vi "P3 E1 RLJ 2015640305.vi"() -> ()   [LabVIEW 2016]
doc: "practica 3: ESTRUCTURAS DE CONTROL\nEjercicio 1 (Cajero automatico).\nNOMBRE DEL ARCHIVO: P3 E1 RLJ 2015640305.vi.\nALUMNO:Ramirez Lopez Jesus Alberto"
uses:
  State.ctl
  Data.ctl
  Control 3.ctl
panel:
  in  "IR A MENU":bool
  in  "Exit":bool
  out "Tab":T1(tab)
  in  "id":bool
  out "Boolean":bool
  out "Pict Ring":i32(ring)
  in  "ok":bool
  in  "0":bool
  in  "8":bool
  in  "9":bool
  in  "7":bool
  in  "6":bool
  in  "5":bool
  in  "4":bool
  in  "3":bool
  in  "2":bool
  in  "1":bool
  out "concatenated string 2":string
  in  "s 2":bool
  out "String 3":string
  in  "edo de cuenta":bool
  in  "deposito oc":bool
  in  "donativo":bool
  in  "pago de tiempo aire":bool
  in  "pago de tarjeta":bool
  in  "retiro":bool
  in  "SALIR":bool
  in  "ingresar":bool
  out "String":string
  in  "Numeric Control 2":dbl
  in  "abonar":bool
  in  "Numeric Control":dbl
  out "String 2":string
  out "Array 2":bool[](array[boolean])
  in  "100":bool
  in  "200":bool
  in  "300":bool
  in  "500":bool
  out "String 4":string
  in  "CDH Tepeyac":bool
  in  "CILAS":bool
  in  "ALAMPYME":bool
  in  "nicolasa":bool
  out "String 6":string
  in  "pedro":bool
  in  "juan":bool
  out "concate":string
  in  "ok 2":bool
  in  "s 3":bool
  in  "1 2":bool
  in  "2 2":bool
  in  "3 2":bool
  in  "4 2":bool
  in  "5 2":bool
  in  "6 2":bool
  in  "7 2":bool
  in  "9 2":bool
  in  "8 2":bool
  in  "0 2":bool
  out "String 7":string
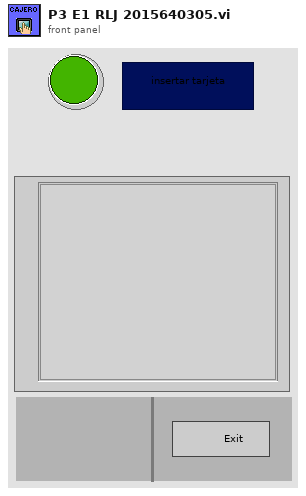
[diagram p1: front panel]
types:
  T1 = enum32{"Page 1", "Page 2", "Page 3", "Page 4", "Page 5", "Page 6", "Page 7", "Page 8", "Page 9", "Page 10"}
  T2 = typedef "Data.ctl" = cluster{"true/false":bool, "String 1":string, "saldo":dbl, "deuda":dbl, "id":bool, "pag1":bool, "seleccion":bool, "edo de cuentas":string, "cuenta error":dbl}
  T3 = typedef "State.ctl" = enum16{"Initialize", "Wait for Event", "id", "contraseña", "error", "retiro de efectivo", "pago de tarjeta", "compra de tiempo aire", "estado de cuenta", "donativo", "deposito a otra cuentas", "teclado", "menu", "Exit"}
  T4 = typedef "Control 3.ctl" = enum32{"Page 1", "Page 2", "Page 3", "Page 4", "Page 5", "Page 6", "Page 7", "Page 8", "Page 9", "Page 10"}
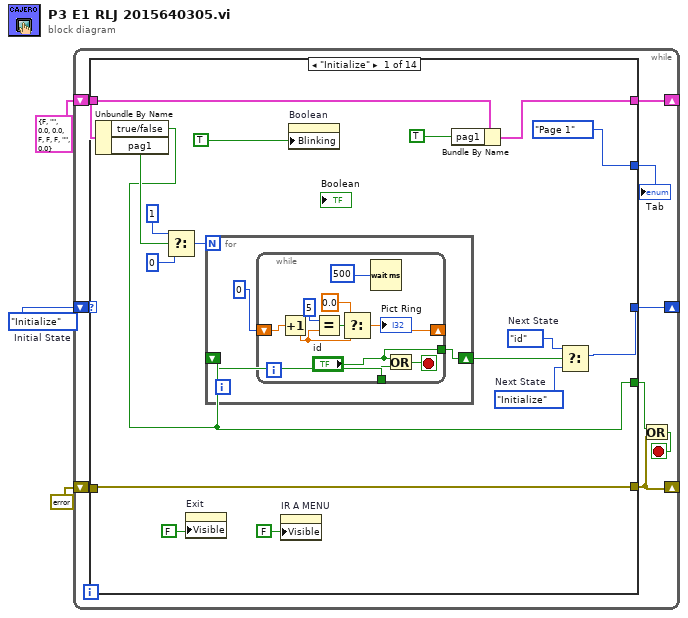
[diagram p0: block diagram]
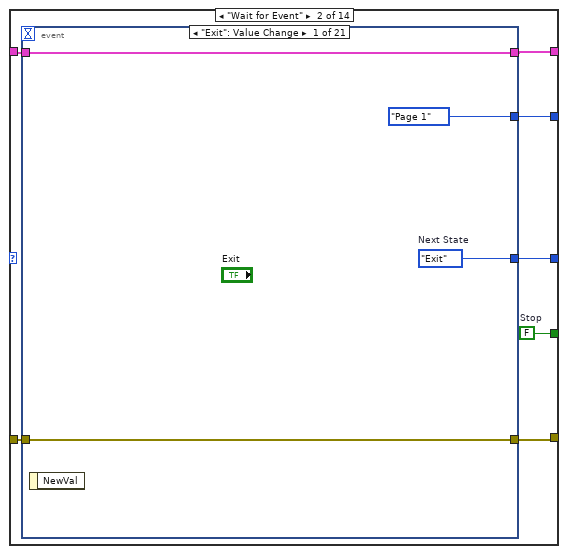
[diagram p2: hidden frame]
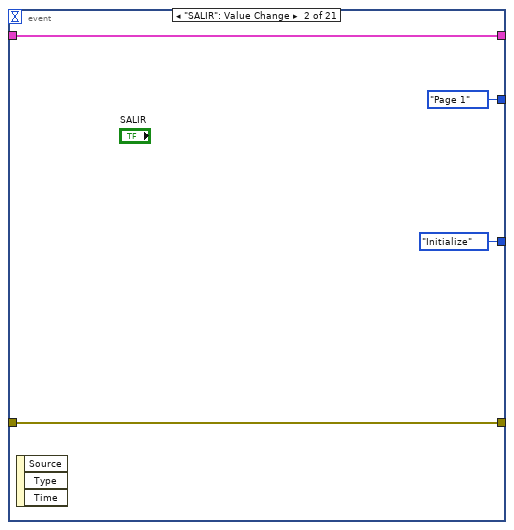
[diagram p3: hidden frame]
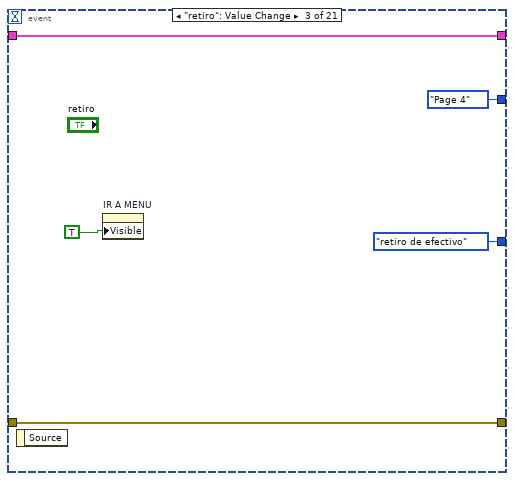
[diagram p4: hidden frame]
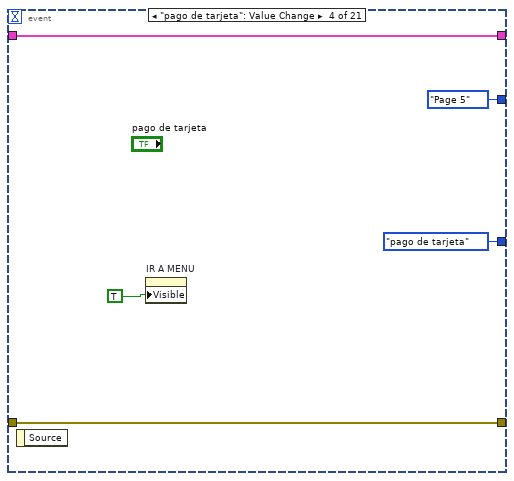
[diagram p5: hidden frame]
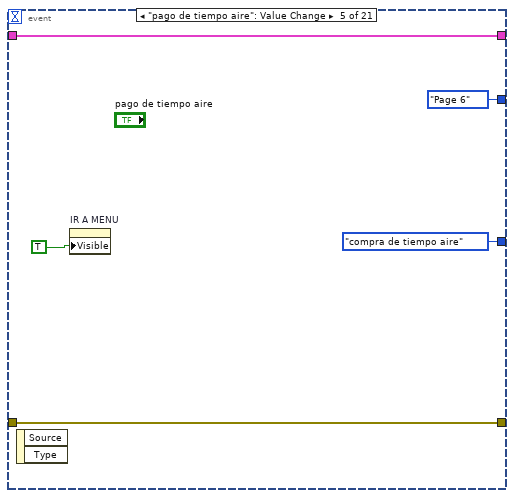
[diagram p6: hidden frame]
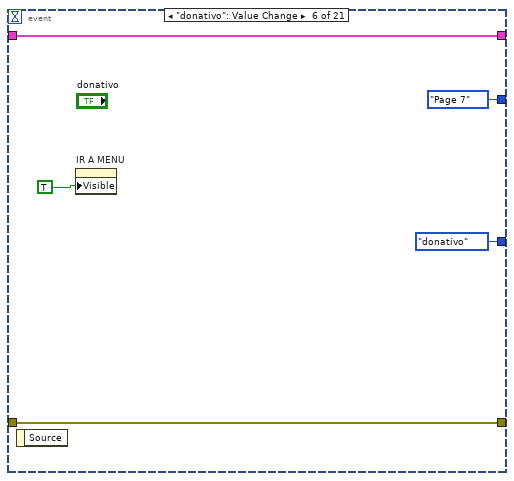
[diagram p7: hidden frame]
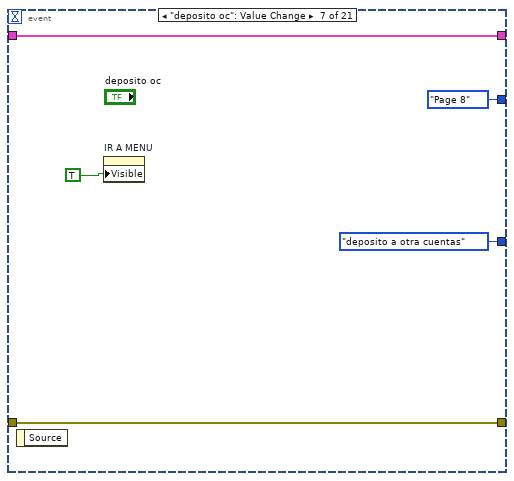
[diagram p8: hidden frame]
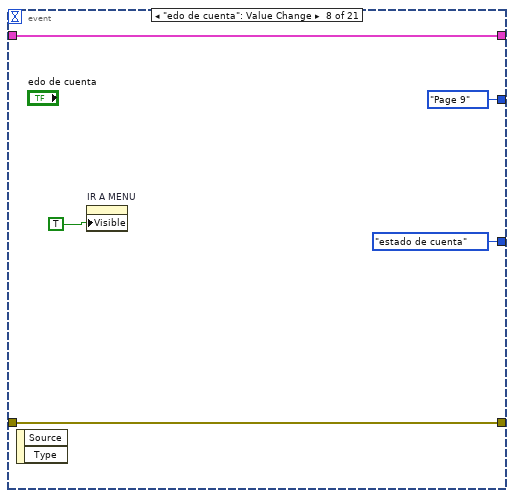
[diagram p9: hidden frame]
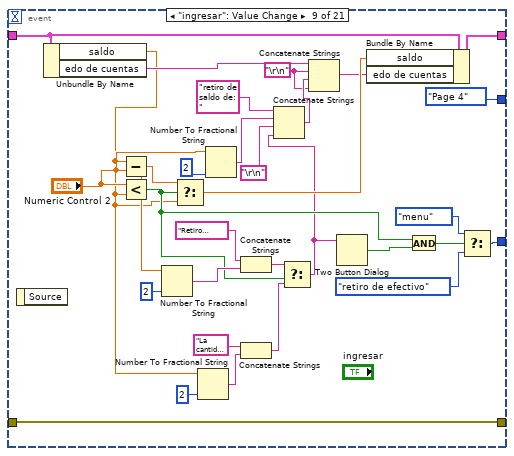
[diagram p10: hidden frame]
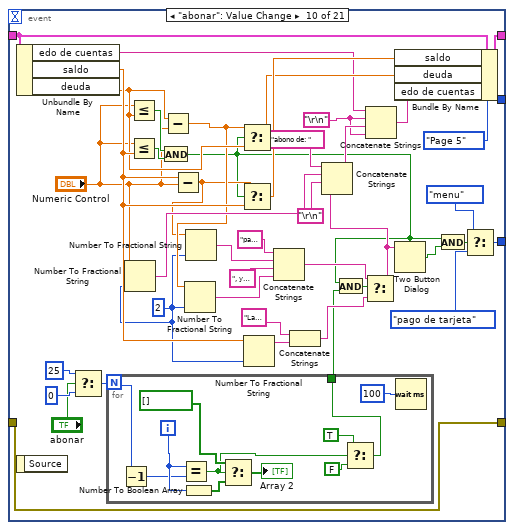
[diagram p11: hidden frame]
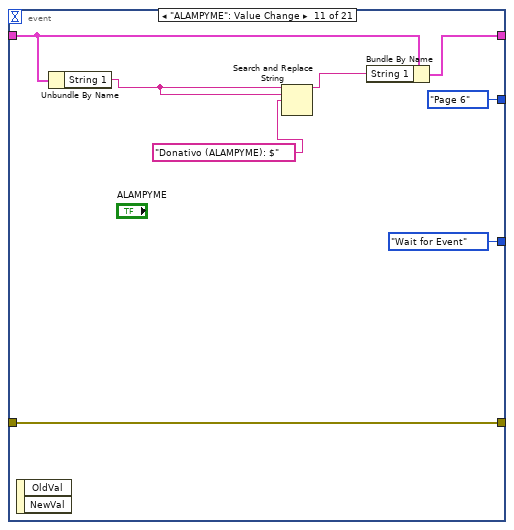
[diagram p12: hidden frame]
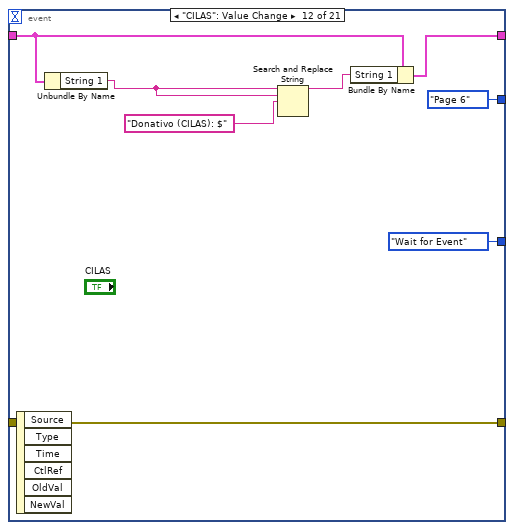
[diagram p13: hidden frame]
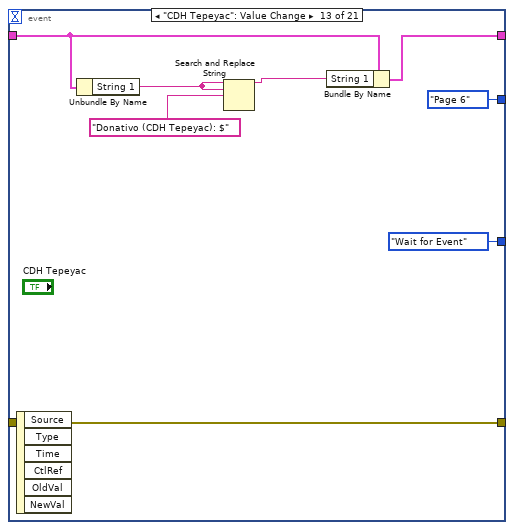
[diagram p14: hidden frame]
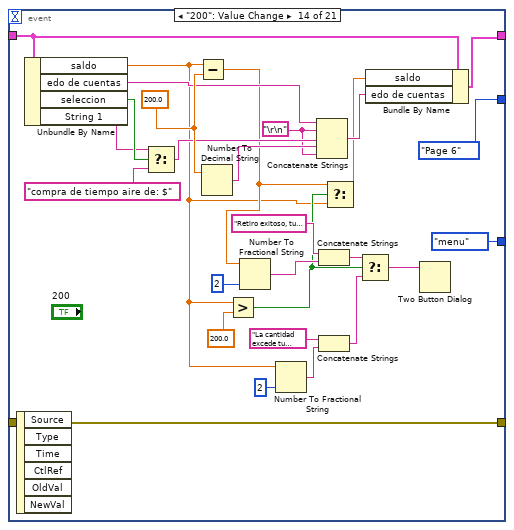
[diagram p15: hidden frame]
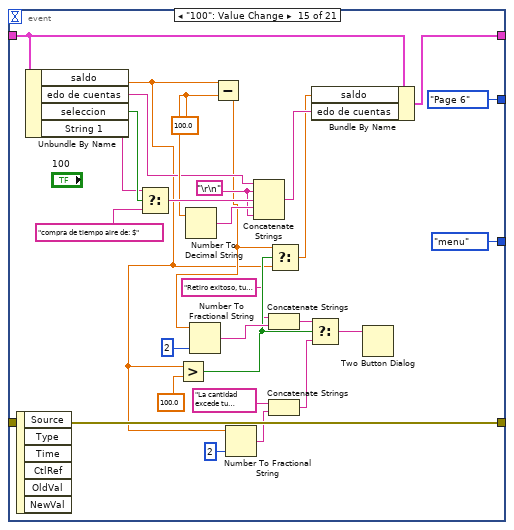
[diagram p16: hidden frame]
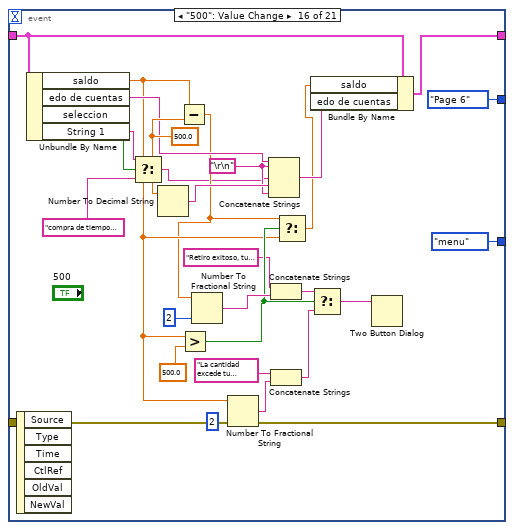
[diagram p17: hidden frame]
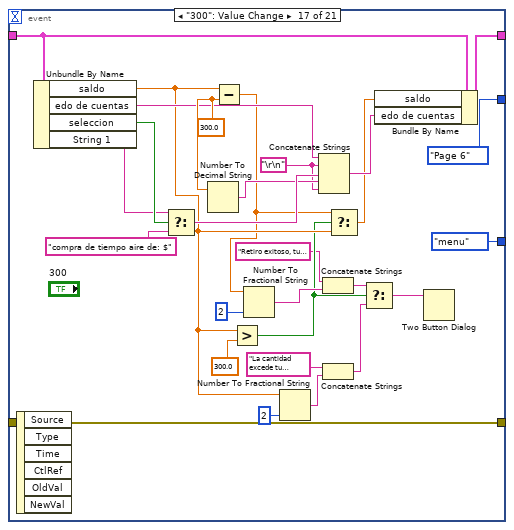
[diagram p18: hidden frame]
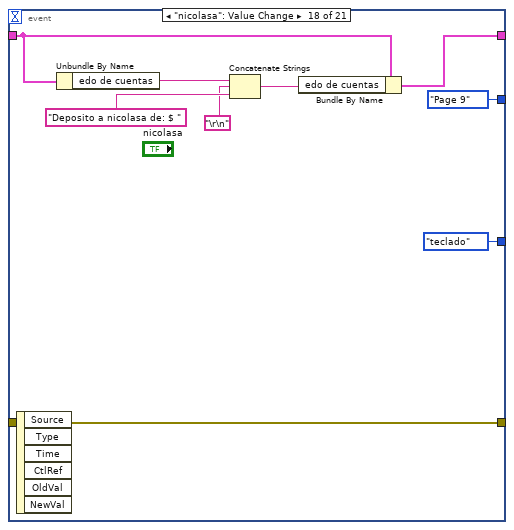
[diagram p19: hidden frame]
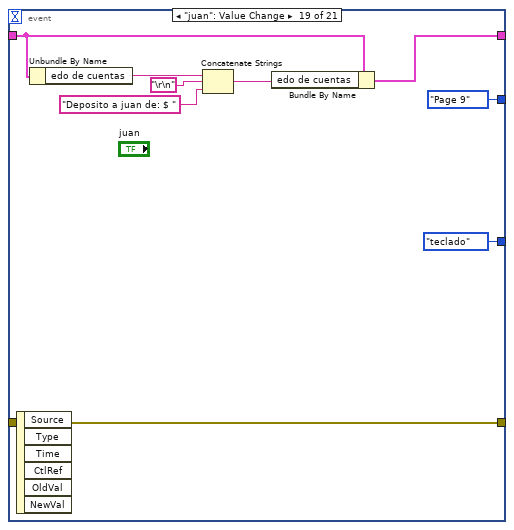
[diagram p20: hidden frame]
diagram:
  w1 = State."Initialize"  # Initial State
  n1 = while {
    shift-right: [w11] -> _
    shift-left: w1 -> [w12]
    shift-right: [w6] -> _
    shift-left: T2 {"true/false"=FALSE, "String 1"="", "saldo"=0.0, "deuda"=0.0, "id"=FALSE, "pag1"=FALSE, "seleccion"=FALSE, "edo de cuentas"="", "cuenta error"=0.0} ("Data") -> [w10]
    shift-right: [w4] -> _
    shift-left: errorcluster {"status"=FALSE, "code"=0, "source"=""} ("error constant") -> [w9]
    stop <- w8 stop-if-true
    # "Main VI State Machine"
    n2 = case shown="\"Initialize\"" w12 {
      tunnel: [w28 w49 w343 w372 w392 State."Wait for Event" ("(Value Not Used)") State."Wait for Event" ("(Value Not Used)") State."Wait for Event" ("(Value Not Used)") State."Wait for Event" ("(Value Not Used)") State."Wait for Event" ("(Value Not Used)") w483 State."Wait for Event" ("(Value Not Used)") State."Wait for Event" ("(Value Not Used)") State."Initialize" ("(Value Not Used)")] -> w11
      tunnel: [w13 w48 FALSE ("Stop Loop?") FALSE ("Stop Loop?") FALSE ("Stop Loop?") FALSE ("Stop Loop?") FALSE ("Stop Loop?") FALSE ("Stop Loop?") FALSE ("Stop Loop?") FALSE ("Stop Loop?") FALSE ("Stop Loop?") FALSE ("Stop Loop?") FALSE ("Stop Loop?") TRUE ("Stop Loop?")] -> w5
      tunnel: w10 -> [w18 w47 w341 w370 w384 w414 w424 w434 w450 w455 w486 w504 w513 w530]
      tunnel: [w17 w46 w341 w371 w383 w414 w424 w434 w449 w455 w487 w504 w521 w530] -> w6
      tunnel: w9 -> [w29 w45 w348 w378 w397 w417 w428 w446 w454 w467 w490 w511 w525 w529]
      tunnel: [w29 w44 w348 w378 w397 w417 w428 w446 w454 w467 w490 w511 w525 w529] -> w4
      tunnel: [Control_3."Page 1" ("Tab Control") w43 Control_3."Page 2" ("Tab Control") w368 w388 Control_3."Page 3" ("Tab Control") Control_3."Page 4" ("Tab Control") Control_3."Page 5" ("Tab Control") Control_3."Page 6" ("Tab Control") Control_3."Page 8" ("Tab Control") Control_3."Page 9" ("Tab Control") Control_3."Page 10" ("Tab Control") Control_3."Page 7" ("Tab Control") Control_3."Page 1" ("Tab Control")] -> w7
      frame "Initialize" {
        w26 = State."Initialize"  # Next State
        w27 = State."id"  # Next State
        # "Initialize - Initialize the application."
        n3 = Unbundle By Name(w18) -> ("true/false"=w13:bool, "pag1"=w14:bool)
        n4 = Select(t=1, s=w14, f=0) -> (s? t:f=w21:i32)
        n5 = property on="Exit" class="Bool"("Visible"=FALSE) -> ()  [unwired: 2 in, 2 out]
        n6 = for {
          N: w21 -> [_]
          shift-right: [w30] -> w22
          shift-left: w13 -> [w31]
          n7 = while {
            shift-right: [w39] -> _
            shift-left: 0 -> [w41]
            tunnel: w31 -> [w34]
            tunnel: ["id"] -> w30
            stop <- w35 stop-if-true
            n8 = Increment(x=w41) -> (x+1=w36:dbl)
            n9 = Equal?(x=5, y=w36) -> (x = y?=w38:bool)
            n10 = Select(t=0.0, s=w38, f=w36) -> (s? t:f=w39:dbl)
            "Pict Ring" <- w39
            n11 = Wait (ms)(milliseconds to wait=u32 500) -> ()  [unwired: 1 out]
            n12 = Or(x="id", y=w34) -> (x .or. y?=w35:bool)
          }
        }
        n13 = property on="IR A MENU" class="Bool"("Visible"=FALSE) -> ()  [unwired: 2 in, 2 out]
        n14 = property on="Boolean" class="Bool (strict)"("Blinking"=TRUE) -> ()  [unwired: 2 in, 2 out]
        n15 = Bundle By Name(cluster=w18, "pag1"=TRUE ("corrimiento")) -> (w17:T2)
        n16 = Select(t=w27, s=w22, f=w26) -> (s? t:f=w28:T3)
      }
      frame "Wait for Event" {
        w48 = FALSE  # Stop
        n17 = event shown="[0] \"Exit\": Value Change" {
          selector: _ -> [_ _ _ _ _ _ _ _ _ _ _ _ _ _ _ _ _ _ _ _ _]
          dyn-events: _ -> [_ _ _ _ _ _ _ _ _ _ _ _ _ _ _ _ _ _ _ _ _]
          timeout: _ -> [_ _ _ _ _ _ _ _ _ _ _ _ _ _ _ _ _ _ _ _ _]
          tunnel: [w53 State."Initialize" ("f") State."retiro de efectivo" ("f") State."pago de tarjeta" ("f") State."compra de tiempo aire" ("f") State."donativo" ("f") State."deposito a otra cuentas" ("f") State."estado de cuenta" ("f") w108 w145 State."Wait for Event" ("f") State."Wait for Event" ("f") State."Wait for Event" ("f") State."menu" ("f") State."menu" ("f") State."menu" ("f") State."menu" ("f") State."teclado" ("f") State."teclado" ("f") State."teclado" ("f") State."menu" ("f")] -> w49
          tunnel: w47 -> [w52 w57 w62 w67 w72 w77 w82 w87 w104 w147 w175 w180 w188 w220 w248 w253 w304 w311 w321 w329 w338]
          tunnel: [w52 w57 w62 w67 w72 w77 w82 w87 w101 w146 w178 w186 w194 w219 w247 w276 w303 w310 w322 w328 w338] -> w46
          tunnel: w45 -> [w51 w56 w61 w66 w71 w76 w81 w86 w118 w160 w179 w187 w195 w223 w251 w279 w307 w316 w325 w334 w337]
          tunnel: [w51 w56 w61 w66 w71 w76 w81 w86 w118 w160 w179 w187 w195 w223 w251 w279 w307 w316 w325 w334 w337] -> w44
          tunnel: [Control_3."Page 1" ("Tab Control") Control_3."Page 1" ("Tab Control") Control_3."Page 4" ("Tab Control") Control_3."Page 5" ("Tab Control") Control_3."Page 6" ("Tab Control") Control_3."Page 7" ("Tab Control") Control_3."Page 8" ("Tab Control") Control_3."Page 9" ("Tab Control") Control_3."Page 4" ("Tab Control") Control_3."Page 5" ("Tab Control") Control_3."Page 6" ("Tab Control") Control_3."Page 6" ("Tab Control") Control_3."Page 6" ("Tab Control") Control_3."Page 6" ("Tab Control") Control_3."Page 6" ("Tab Control") Control_3."Page 6" ("Tab Control") Control_3."Page 6" ("Tab Control") Control_3."Page 9" ("Tab Control") Control_3."Page 9" ("Tab Control") Control_3."Page 9" ("Tab Control") Control_3."Page 3" ("Tab Control")] -> w43
          event "Exit": Value Change {
            w53 = State."Exit"  # Next State
            n18 = event-data() -> ()  [unwired: 1 in, 1 out]
          }
          event "SALIR": Value Change {
            n19 = event-data() -> ()  [unwired: 1 in, 3 out]
          }
          event "retiro": Value Change {
            n20 = event-data() -> ()  [unwired: 1 in, 1 out]
            n21 = property on="IR A MENU" class="Bool"("Visible"=TRUE) -> ()  [unwired: 2 in, 2 out]
          }
          event "pago de tarjeta": Value Change {
            n22 = event-data() -> ()  [unwired: 1 in, 1 out]
            n23 = property on="IR A MENU" class="Bool"("Visible"=TRUE) -> ()  [unwired: 2 in, 2 out]
          }
          event "pago de tiempo aire": Value Change {
            n24 = event-data() -> ()  [unwired: 1 in, 2 out]
            n25 = property on="IR A MENU" class="Bool"("Visible"=TRUE) -> ()  [unwired: 2 in, 2 out]
          }
          event "donativo": Value Change {
            n26 = event-data() -> ()  [unwired: 1 in, 1 out]
            n27 = property on="IR A MENU" class="Bool"("Visible"=TRUE) -> ()  [unwired: 2 in, 2 out]
          }
          event "deposito oc": Value Change {
            n28 = event-data() -> ()  [unwired: 1 in, 1 out]
            n29 = property on="IR A MENU" class="Bool"("Visible"=TRUE) -> ()  [unwired: 2 in, 2 out]
          }
          event "edo de cuenta": Value Change {
            n30 = event-data() -> ()  [unwired: 1 in, 2 out]
            n31 = property on="IR A MENU" class="Bool"("Visible"=TRUE) -> ()  [unwired: 2 in, 2 out]
          }
          event "ingresar": Value Change {
            w93 = "\r\n"
            n32 = event-data() -> ()  [unwired: 1 in, 1 out]
            n33 = Unbundle By Name(w104) -> ("saldo"=w89:dbl, "edo de cuentas"=w100:string)
            n34 = Subtract(x=w89, y="Numeric Control 2") -> (x-y=w117:dbl)
            n35 = Less?(x="Numeric Control 2", y=w89) -> (x < y?=w110:bool)
            n36 = Number To Fractional String(number=w117, precision (6)=i16 2) -> (F-format string=w116:string)  [unwired: 2 in]
            n37 = Select(t=w117, s=w110, f=w89) -> (s? t:f=w103:dbl)
            n38 = Number To Fractional String(number=w89, precision (6)=i16 2) -> (F-format string=w113:string)  [unwired: 2 in]
            n39 = Number To Fractional String(number="Numeric Control 2", precision (6)=i16 2) -> (F-format string=w98:string)  [unwired: 2 in]
            n40 = Concatenate Strings("Retiro exitoso, tu saldo actual es de: \n" ("string"), w116) -> (w115:string)
            n41 = Concatenate Strings("La cantidad excede tu credito, el cual es de: \n" ("string"), w113) -> (w112:string)
            n42 = Select(t=w115, s=w110, f=w112) -> (s? t:f=w88:string)
            n43 = Concatenate Strings("retiro de saldo de: " ("string"), w98, "\r\n", w88) -> (w96:string)
            n44 = Concatenate Strings(w100, w93, w96, w93) -> (w99:string)
            n45 = Two Button Dialog(message=w88) -> (T button?=w111:bool)  [unwired: 2 in]
            n46 = Bundle By Name(cluster=w104, "saldo"=w103, "edo de cuentas"=w99) -> (w101:T2)
            n47 = And(x=w110, y=w111) -> (x .and. y?=w109:bool)
            n48 = Select(t=State."menu" ("Next State"), s=w109, f=State."retiro de efectivo") -> (s? t:f=w108:T3)
          }
          event "abonar": Value Change {
            w122 = i16 2 ("precision (6)")
            w126 = "\r\n"
            n49 = Unbundle By Name(w147) -> ("edo de cuentas"=w133:string, "saldo"=w154:dbl, "deuda"=w141:dbl)
            n50 = event-data() -> ()  [unwired: 1 in, 1 out]
            n51 = Select(t=25, s="abonar", f=0) -> (s? t:f=w137:i32)
            n52 = for {
              N: w137 -> [w169]
              tunnel: [w161] -> w119
              i -> [w170]
              n53 = Decrement(x=w169) -> (x-1=w168:i32)
              n54 = Equal?(x=w170, y=w168) -> (x = y?=w164:bool)
              n55 = Number To Boolean Array(number=w170) -> (Boolean array=w167:bool[])
              n56 = Select(t=bool[] [], s=w164, f=w167) -> (s? t:f=→"Array 2":bool[])
              n57 = Select(t=TRUE, s=w164, f=FALSE) -> (s? t:f=w161:bool)
              n58 = Wait (ms)(milliseconds to wait=u32 100) -> ()  [unwired: 1 out]
            }
            n59 = Number To Fractional String(number="Numeric Control", precision (6)=w122) -> (F-format string=w130:string)  [unwired: 2 in]
            n60 = Less Or Equal?(x="Numeric Control", y=w141) -> (x <= y?=w144:bool)
            n61 = Less Or Equal?(x="Numeric Control", y=w154) -> (x <= y?=w143:bool)
            n62 = And(x=w144, y=w143) -> (x .and. y?=w120:bool)
            n63 = Subtract(x=w141, y="Numeric Control") -> (x-y=w123:dbl)
            n64 = Subtract(x=w154, y="Numeric Control") -> (x-y=w121:dbl)
            n65 = Number To Fractional String(number=w123, precision (6)=w122) -> (F-format string=w125:string)  [unwired: 2 in]
            n66 = Number To Fractional String(number=w121, precision (6)=w122) -> (F-format string=w159:string)  [unwired: 2 in]
            n67 = Select(t=w123, s=w120, f=w141) -> (s? t:f=w142:dbl)
            n68 = Select(t=w121, s=w120, f=w154) -> (s? t:f=w148:dbl)
            n69 = Number To Fractional String(number=w154, precision (6)=w122) -> (F-format string=w156:string)  [unwired: 2 in]
            n70 = Concatenate Strings("pago exitoso, tu saldo actual es de: \n" ("string"), w159, ", y tienes un adeudo de: " ("string"), w125) -> (w158:string)
            n71 = Concatenate Strings("La cantidad excede tu credito, el cual es de: \n" ("string"), w156) -> (w155:string)
            n72 = And(x=w120, y=w119) -> (x .and. y?=w135:bool)
            n73 = Select(t=w158, s=w135, f=w155) -> (s? t:f=w128:string)
            n74 = Concatenate Strings("abono de: " ("string"), w130, "\r\n", w128) -> (w129:string)
            n75 = Concatenate Strings(w133, w126, w129, w126) -> (w134:string)
            n76 = Bundle By Name(cluster=w147, "saldo"=w148, "deuda"=w142, "edo de cuentas"=w134) -> (w146:T2)
            n77 = Two Button Dialog(message=w128) -> (T button?=w153:bool)  [unwired: 2 in]
            n78 = And(x=w120, y=w153) -> (x .and. y?=w152:bool)
            n79 = Select(t=State."menu" ("Next State"), s=w152, f=State."pago de tarjeta") -> (s? t:f=w145:T3)
          }
          event "ALAMPYME": Value Change {
            n80 = event-data() -> ()  [unwired: 1 in, 2 out]
            n81 = Unbundle By Name(w175) -> ("String 1"=w174:string)
            n82 = Search and Replace String(input string=w174, search string=w174, replace string="Donativo (ALAMPYME): $" ("String <Replace Me>")) -> (result string=w172:string)  [unwired: 5 in, 3 out]
            n83 = Bundle By Name(cluster=w175, "String 1"=w172) -> (w178:T2)
          }
          event "CILAS": Value Change {
            n84 = event-data() -> ()  [unwired: 1 in, 6 out]
            n85 = Unbundle By Name(w180) -> ("String 1"=w183:string)
            n86 = Search and Replace String(input string=w183, search string=w183, replace string="Donativo (CILAS): $" ("String <Replace Me>")) -> (result string=w182:string)  [unwired: 5 in, 3 out]
            n87 = Bundle By Name(cluster=w180, "String 1"=w182) -> (w186:T2)
          }
          event "CDH Tepeyac": Value Change {
            n88 = event-data() -> ()  [unwired: 1 in, 6 out]
            n89 = Unbundle By Name(w188) -> ("String 1"=w191:string)
            n90 = Search and Replace String(input string=w191, search string=w191, replace string="Donativo (CDH Tepeyac): $" ("String <Replace Me>")) -> (result string=w189:string)  [unwired: 5 in, 3 out]
            n91 = Bundle By Name(cluster=w188, "String 1"=w189) -> (w194:T2)
          }
          event "200": Value Change {
            w210 = "\r\n"
            w218 = 200.0 ("y")
            n92 = event-data() -> ()  [unwired: 1 in, 6 out]
            n93 = Unbundle By Name(w220) -> ("saldo"=w197:dbl, "edo de cuentas"=w211:string, "seleccion"=w216:bool, "String 1"=w212:string)
            n94 = Select(t=w212, s=w216, f="compra de tiempo aire de: $") -> (s? t:f=w214:string)
            n95 = Subtract(x=w197, y=w218) -> (x-y=w198:dbl)
            n96 = Number To Decimal String(number=w218) -> (decimal integer string=w213:string)  [unwired: 1 in]
            n97 = Greater?(x=w197, y=200.0) -> (0:w199:bool)
            n98 = Number To Fractional String(number=w198, precision (6)=i16 2) -> (F-format string=w209:string)  [unwired: 2 in]
            n99 = Number To Fractional String(number=w197, precision (6)=i16 2) -> (F-format string=w206:string)  [unwired: 2 in]
            n100 = Concatenate Strings(w211, w210, w214, w213, w210) -> (w217:string)
            n101 = Concatenate Strings("Retiro exitoso, tu saldo actual es de: \n" ("string"), w209) -> (w208:string)
            n102 = Concatenate Strings("La cantidad excede tu credito, el cual es de: \n" ("string"), w206) -> (w205:string)
            n103 = Select(t=w198, s=w199, f=w197) -> (s? t:f=w196:dbl)
            n104 = Select(t=w208, s=w199, f=w205) -> (s? t:f=w202:string)
            n105 = Bundle By Name(cluster=w220, "saldo"=w196, "edo de cuentas"=w217) -> (w219:T2)
            n106 = Two Button Dialog(message=w202) -> ()  [unwired: 2 in, 1 out]
          }
          event "100": Value Change {
            w238 = "\r\n"
            w242 = 100.0 ("y")
            n107 = event-data() -> ()  [unwired: 1 in, 6 out]
            n108 = Unbundle By Name(w248) -> ("saldo"=w225:dbl, "edo de cuentas"=w239:string, "seleccion"=w241:bool, "String 1"=w240:string)
            n109 = Select(t=w240, s=w241, f="compra de tiempo aire de: $") -> (s? t:f=w245:string)
            n110 = Greater?(x=w225, y=100.0) -> (0:w228:bool)
            n111 = Number To Decimal String(number=w242) -> (decimal integer string=w244:string)  [unwired: 1 in]
            n112 = Subtract(x=w225, y=w242) -> (x-y=w226:dbl)
            n113 = Number To Fractional String(number=w226, precision (6)=i16 2) -> (F-format string=w237:string)  [unwired: 2 in]
            n114 = Number To Fractional String(number=w225, precision (6)=i16 2) -> (F-format string=w234:string)  [unwired: 2 in]
            n115 = Concatenate Strings(w239, w238, w245, w244, w238) -> (w243:string)
            n116 = Concatenate Strings("Retiro exitoso, tu saldo actual es de: \n" ("string"), w237) -> (w236:string)
            n117 = Concatenate Strings("La cantidad excede tu credito, el cual es de: \n" ("string"), w234) -> (w233:string)
            n118 = Select(t=w226, s=w228, f=w225) -> (s? t:f=w224:dbl)
            n119 = Select(t=w236, s=w228, f=w233) -> (s? t:f=w231:string)
            n120 = Bundle By Name(cluster=w248, "saldo"=w224, "edo de cuentas"=w243) -> (w247:T2)
            n121 = Two Button Dialog(message=w231) -> ()  [unwired: 2 in, 1 out]
          }
          event "500": Value Change {
            w271 = 500.0 ("y")
            w268 = "\r\n"
            n122 = event-data() -> ()  [unwired: 1 in, 6 out]
            n123 = Unbundle By Name(w253) -> ("saldo"=w257:dbl, "edo de cuentas"=w269:string, "seleccion"=w272:bool, "String 1"=w270:string)
            n124 = Select(t=w270, s=w272, f="compra de tiempo aire de: $") -> (s? t:f=w252:string)
            n125 = Number To Decimal String(number=w271) -> (decimal integer string=w274:string)  [unwired: 1 in]
            n126 = Subtract(x=w257, y=w271) -> (x-y=w256:dbl)
            n127 = Greater?(x=w257, y=500.0) -> (0:w258:bool)
            n128 = Number To Fractional String(number=w256, precision (6)=i16 2) -> (F-format string=w267:string)  [unwired: 2 in]
            n129 = Number To Fractional String(number=w257, precision (6)=i16 2) -> (F-format string=w264:string)  [unwired: 2 in]
            n130 = Concatenate Strings(w269, w268, w252, w274, w268) -> (w273:string)
            n131 = Concatenate Strings("Retiro exitoso, tu saldo actual es de: \n" ("string"), w267) -> (w266:string)
            n132 = Concatenate Strings("La cantidad excede tu credito, el cual es de: \n" ("string"), w264) -> (w263:string)
            n133 = Select(t=w256, s=w258, f=w257) -> (s? t:f=w255:dbl)
            n134 = Bundle By Name(cluster=w253, "saldo"=w255, "edo de cuentas"=w273) -> (w276:T2)
            n135 = Select(t=w266, s=w258, f=w263) -> (s? t:f=w261:string)
            n136 = Two Button Dialog(message=w261) -> ()  [unwired: 2 in, 1 out]
          }
          event "300": Value Change {
            w294 = "\r\n"
            w299 = 300.0 ("y")
            n137 = event-data() -> ()  [unwired: 1 in, 6 out]
            n138 = Unbundle By Name(w304) -> ("saldo"=w284:dbl, "edo de cuentas"=w295:string, "seleccion"=w297:bool, "String 1"=w296:string)
            n139 = Select(t=w296, s=w297, f="compra de tiempo aire de: $") -> (s? t:f=w301:string)
            n140 = Number To Decimal String(number=w299) -> (decimal integer string=w300:string)  [unwired: 1 in]
            n141 = Subtract(x=w284, y=w299) -> (x-y=w282:dbl)
            n142 = Greater?(x=w284, y=300.0) -> (0:w283:bool)
            n143 = Number To Fractional String(number=w282, precision (6)=i16 2) -> (F-format string=w293:string)  [unwired: 2 in]
            n144 = Number To Fractional String(number=w284, precision (6)=i16 2) -> (F-format string=w290:string)  [unwired: 2 in]
            n145 = Concatenate Strings(w295, w294, w301, w300, w294) -> (w298:string)
            n146 = Concatenate Strings("Retiro exitoso, tu saldo actual es de: \n" ("string"), w293) -> (w292:string)
            n147 = Concatenate Strings("La cantidad excede tu credito, el cual es de: \n" ("string"), w290) -> (w289:string)
            n148 = Select(t=w282, s=w283, f=w284) -> (s? t:f=w281:dbl)
            n149 = Select(t=w292, s=w283, f=w289) -> (s? t:f=w287:string)
            n150 = Bundle By Name(cluster=w304, "saldo"=w281, "edo de cuentas"=w298) -> (w303:T2)
            n151 = Two Button Dialog(message=w287) -> ()  [unwired: 2 in, 1 out]
          }
          event "nicolasa": Value Change {
            n152 = event-data() -> ()  [unwired: 1 in, 6 out]
            n153 = Unbundle By Name(w311) -> ("edo de cuentas"=w312:string)
            n154 = Concatenate Strings(w312, "\r\n", "Deposito a nicolasa de: $ " ("string")) -> (w313:string)
            n155 = Bundle By Name(cluster=w311, "edo de cuentas"=w313) -> (w310:T2)
          }
          event "juan": Value Change {
            n156 = event-data() -> ()  [unwired: 1 in, 6 out]
            n157 = Unbundle By Name(w321) -> ("edo de cuentas"=w320:string)
            n158 = Concatenate Strings(w320, "\r\n", "Deposito a juan de: $ " ("string")) -> (w319:string)
            n159 = Bundle By Name(cluster=w321, "edo de cuentas"=w319) -> (w322:T2)
          }
          event "pedro": Value Change {
            n160 = event-data() -> ()  [unwired: 1 in, 6 out]
            n161 = Unbundle By Name(w329) -> ("edo de cuentas"=w330:string)
            n162 = Concatenate Strings(w330, "\r\n", "Deposito a pedro de: $ " ("string")) -> (w331:string)
            n163 = Bundle By Name(cluster=w329, "edo de cuentas"=w331) -> (w328:T2)
          }
          event "IR A MENU": Value Change {
            n164 = event-data() -> ()  [unwired: 1 in, 2 out]
          }
        }
      }
      frame "contraseña" {
        w344 = State."error"  # Next State
        w345 = State."menu"  # Next State
        n165 = while {
          tunnel: [w351] -> w339
          stop <- "ok" stop-if-true
          n166 = call "tableronum.vi"("1"="1", "8"="8", "OK"="ok", "3"="3", "2"="2", "s 2"="s 2", "4"="4", "5"="5", "6"="6", "0"="0", "7"="7", "9"="9") -> ("concatenated string"=w351:string)  [unwired: 3 in]
          "concatenated string 2" <- w351
        }
        n167 = Unbundle By Name(w341) -> ()  [unwired: 1 out]
        n168 = Equal?(x=w339, y="1393") -> (x = y?=w342:bool)
        n169 = Select(t=w345, s=w342, f=w344) -> (s? t:f=w343:T3)
      }
      frame "error" {
        n170 = Unbundle By Name(w370) -> ("cuenta error"=w369:dbl)
        n171 = Increment(x=w369) -> (x+1=w376:dbl)
        n172 = Equal?(x=w376, y=3.0) -> (x = y?=w365:bool)
        n173 = Bundle By Name(cluster=w370, "cuenta error"=w376, "true/false"=w365) -> (w371:T2)
        n174 = Select(t="Cancelación de sesión" ("message"), s=w365, f="error" ("message")) -> (s? t:f=w362:string)
        n175 = One Button Dialog(message=w362) -> ()  [unwired: 1 in, 1 out]
        n176 = Select(t=Control_3."Page 1" ("Tab Control"), s=w365, f=Control_3."Page 2" ("Tab Control")) -> (s? t:f=w368:T4)
        n177 = Select(t=State."Initialize" ("(Value Not Used)"), s=w365, f=State."contraseña" ("(Value Not Used)")) -> (s? t:f=w372:T3)
      }
      frame "id" {
        w393 = State."Initialize"  # Initial State
        w394 = State."contraseña"  # Initial State
        # "User State 1 - Replace this state with functionality for your own application."
        n178 = Random Number (0-1)() -> (number: 0 to 1=w385:dbl)
        n179 = Random Number (0-1)() -> (number: 0 to 1=w386:dbl)
        n180 = expression code="6000-(1000*x)"(w385) -> (w382:dbl)
        n181 = expression code="10000-(6000*x)"(w386) -> (w380:dbl)
        n182 = To Quad Integer(1:w382) -> (0:w381:i64)
        n183 = To Quad Integer(1:w380) -> (0:w379:i64)
        n184 = Bundle By Name(cluster=w384, "saldo"=w381, "deuda"=w379) -> (w383:T2)
        n185 = Two Button Dialog(message="Es usted RAMIREZ LOPEZ JESUS ALBERTO\nCON NUMERO DE BOLETA 2015640305" ("Running User State 1"), 1:"no" ("F button name (\"Cancel\")"), 2:"si" ("T button name (\"OK\")")) -> (T button?=w390:bool)
        n186 = Select(t=w394, s=w390, f=w393) -> (s? t:f=w392:T3)
        n187 = Select(t=Control_3."Page 2" ("Tab Control"), s=w390, f=Control_3."Page 1" ("Tab Control")) -> (s? t:f=w388:T4)
      }
      frame "menu" {
        n188 = Unbundle By Name(w414) -> ("saldo"=w407:dbl, "deuda"=w401:dbl)
        n189 = property on="Exit" class="Bool"("Visible"=TRUE) -> ()  [unwired: 2 in, 2 out]
        n190 = property on="IR A MENU" class="Bool"("Visible"=FALSE) -> ()  [unwired: 2 in, 2 out]
        n191 = Number To Fractional String(number=w401, precision (6)=i16 2) -> (F-format string=w405:string)  [unwired: 2 in]
        n192 = Number To Fractional String(number=w407, precision (6)=i16 2) -> (F-format string=w412:string)  [unwired: 2 in]
        n193 = Concatenate Strings("TU SALDO ES DE:   " ("message"), w412) -> (w409:string)
        n194 = Concatenate Strings("TU DEUDA ES DE:   " ("message"), w405) -> (w408:string)
        n195 = Concatenate Strings(w409, "\r\n", w408) -> (→"String 3":string)
      }
      frame "retiro de efectivo" {
        n196 = Unbundle By Name(w424) -> ("saldo"=w419:dbl)
        n197 = Number To Fractional String(number=w419, precision (6)=i16 2) -> (F-format string=w423:string)  [unwired: 2 in]
        n198 = Concatenate Strings("RETIRO DE EFECTIVO:    \n tu credito es de: " ("string"), w423, "\nIngresa el valor a retirar" ("string")) -> (→"String":string)
      }
      frame "pago de tarjeta" {
        n199 = Unbundle By Name(w434) -> ("saldo"=w439:dbl)
        n200 = Unbundle By Name(w434) -> ("deuda"=w435:dbl)
        n201 = Number To Fractional String(number=w439, precision (6)=i16 2) -> (F-format string=w442:string)  [unwired: 2 in]
        n202 = Number To Fractional String(number=w435, precision (6)=i16 2) -> (F-format string=w438:string)  [unwired: 2 in]
        n203 = Concatenate Strings("PAGO DE TARJETA:    \n tu credito es de: " ("string"), w442, "\nIngresa el valor a retirar" ("string")) -> (w433:string)
        n204 = Concatenate Strings("\nsu adeudo de tarjeta de credito es de: " ("string"), w438, "\nIngresa el valor a abonar" ("string")) -> (w432:string)
        n205 = Concatenate Strings(w433, w432) -> (→"String 2":string)
      }
      frame "compra de tiempo aire" {
        n206 = Bundle By Name(cluster=w450, "String 1"="COMPRA DE TIEMPO AIRE\nselecciona el valor de tu recarga" ("String <Replace Me>"), "seleccion"=FALSE) -> (w449:T2)
      }
      frame "deposito a otra cuentas" {
        w456 = "\r\n"
        n207 = Unbundle By Name(w455) -> ("saldo"=w462:dbl)
        n208 = Number To Fractional String(number=w462, precision (6)=i16 2) -> (F-format string=w459:string)  [unwired: 2 in]
        n209 = Concatenate Strings("DEPOSITO A OTRAS CUENTAS" ("string"), w456, "Tu saldo es de: " ("string"), w456, w459, w456, "Selecciona la persona a la que realizaras el deposito:") -> (→"String 6":string)
      }
      frame "teclado" {
        w471 = "\r\n"
        n210 = while {
          tunnel: [w503] -> w473
          tunnel: ["ok 2"] -> w482
          stop <- "ok 2" stop-if-true
          n211 = call "tableronum.vi"("1"="1 2", "8"="8 2", "OK"="ok 2", "3"="3 2", "2"="2 2", "s 2"="s 3", "4"="4 2", "5"="5 2", "6"="6 2", "0"="0 2", "7"="7 2", "9"="9 2") -> ("concatenated string"=w503:string)  [unwired: 3 in]
          "concate" <- w503
        }
        n212 = property on="IR A MENU" class="Bool"("Visible"=FALSE) -> ()  [unwired: 2 in, 2 out]
        n213 = Unbundle By Name(w486) -> ("saldo"=w478:dbl, "edo de cuentas"=w474:string)
        n214 = property on="Exit" class="Bool"("Visible"=FALSE) -> ()  [unwired: 2 in, 2 out]
        n215 = Fract/Exp String To Number(string=w473) -> (number=w481:dbl)  [unwired: 3 in, 1 out]
        n216 = Subtract(x=w478, y=w481) -> (x-y=w479:dbl)
        n217 = Less Or Equal?(x=w481, y=w478) -> (x <= y?=w477:bool)
        n218 = Select(t=w479, s=w477, f=w478) -> (s? t:f=w480:dbl)
        n219 = Select(t="transaccion exitosa", s=w477, f="cantidad incorrecta") -> (s? t:f=w472:string)
        n220 = Concatenate Strings(w474, w473, w471, w472, w471) -> (w470:string)
        n221 = Bundle By Name(cluster=w486, "saldo"=w480, "edo de cuentas"=w470) -> (w487:T2)
        n222 = One Button Dialog(message=w472) -> ()  [unwired: 1 in, 1 out]
        n223 = Select(t=State."menu" ("(Value Not Used)"), s=w482, f=State."teclado" ("(Value Not Used)")) -> (s? t:f=w483:T3)
      }
      frame "estado de cuenta" {
        n224 = Unbundle By Name(w504) -> ("edo de cuentas"=w505:string)
        n225 = Concatenate Strings("ESTADO DE CUENTA" ("string"), w505) -> (→"String 7":string)
      }
      frame "donativo" {
        w516 = "\r\n"
        w515 = "DONATIVO\nselecciona la asociacion a la que quieras donar" ("String <Replace Me>")
        n226 = Unbundle By Name(w513) -> ("saldo"=w512:dbl)
        n227 = Number To Fractional String(number=w512, precision (6)=i16 2) -> (F-format string=w517:string)  [unwired: 2 in]
        n228 = Bundle By Name(cluster=w513, "String 1"=w515, "seleccion"=TRUE) -> (w521:T2)
        n229 = Concatenate Strings(w515, w516, "Tu saldo es de: " ("string"), w516, w517, w516) -> (→"String 4":string)
      }
      frame "Exit" {
      }
    }
    "Tab" <- w7
    n230 = Or(x=w5, y=w4) -> (x .or. y?=w8:bool)
  }
